vi "Finish.vi"   [LabVIEW 2013]
doc: "This VI is called just before exiting. It is expected to close I/O refnum, save collected data, etc."
uses:
  <vilib>/Rock Robotics/WPI/Joystick/WPI_JoystickGetSetRefNum.vi
types:
  T1 = typedef "WPI_MotorControlDeviceRef.ctl" = cluster{"DeviceStatus":errorcluster, "Type":enum16{"PWM", "CAN"}, "PWM":cluster{"Digital Module":T2, "PWM Channel":T3, "DeadBand":T4}, "CAN":cluster{"Device Number":u8, "Control Mode":T5, "Semaphore":T6, "Max Vout":dbl}, "Invert":bool, "TransformRef":T7, "InvTransformRef":T7}
  T2 = typedef "FPGA_TypedefDigitalModule.ctl" = enum16{"Digital Module 1", "Digital Module 2"}
  T3 = typedef "FPGA_DIOPWMChannel.ctl" = enum8{"PWM 1", "PWM 2", "PWM 3", "PWM 4", "PWM 5", "PWM 6", "PWM 7", "PWM 8", "PWM 9", "PWM 10", "Invalid"}
  T4 = typedef "WPI_PWMDeadband.ctl" = cluster{"Name":string, "maxPositivePwm":i32, "minPositivePwm":i32, "centerPwm":i32, "maxNegativePwm":i32, "minNegativePwm":i32, "angularRange":u16}
  T5 = typedef "WPI_CANJaguar_ControlMode.ctl" = enum8{"Percent VBus", "Current", "Speed", "Position", "Voltage"}
  T6 = typedef "Semaphore RefNum" = refnum<k1>
  T7 = typedef "WPI_PWMTransform_ConPane.ctl" = refnum<vi>
  T8 = typedef "WPI_SolenoidDevRef.ctl" = cluster{"DevStatus":errorcluster, "Solenoid Module":T9, "Forward Solenoid Channel":T10, "Reverse Solenoid Channel":T10}
  T9 = typedef "FPGA_TypedefSolenoidModule.ctl" = enum16{"Solenoid Module 1", "Solenoid Module 2"}
  T10 = typedef "WPI_SolenoidChannel.ctl" = enum8{"Solenoid 1", "Solenoid 2", "Solenoid 3", "Solenoid 4", "Solenoid 5", "Solenoid 6", "Solenoid 7", "Solenoid 8", "Invalid"}
  T11 = typedef "WPI_DigitalInputDevRef.ctl" = cluster{"DevStatus":errorcluster, "DIO Channel":T12, "Digital Module":T2}
  T12 = typedef "FPGA_DIOChannel.ctl" = enum8{"DIO 1", "DIO 2", "DIO 3", "DIO 4", "DIO 5", "DIO 6", "DIO 7", "DIO 8", "DIO 9", "DIO 10", "DIO 11", "DIO 12", "DIO 13", "DIO 14", "Invalid"}
  T13 = typedef "WPI_CameraDevRef.ctl" = cluster{"Camera Address":string, "CameraStatus":errorcluster, "Acquire Image Notifier":refnum<notifier>}
  T14 = typedef "WPI_JoystickDevRef.ctl" = cluster{"Device":T15}
  T15 = typedef "WPI_JoystickDeviceEnum.ctl" = enum16{"USB 1", "USB 2", "USB 3", "USB 4", "Kinect 1", "Kinect 2"}
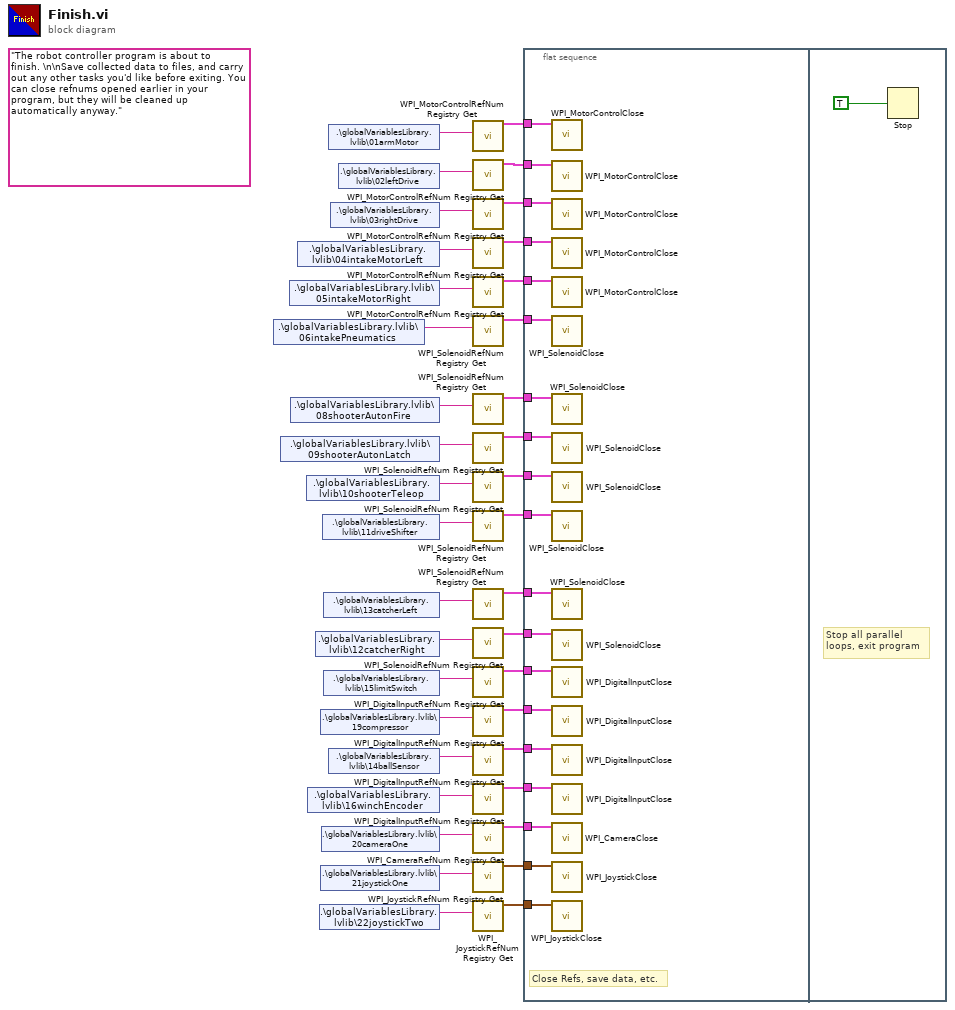
[diagram p0: block diagram]
diagram:
  (unwired) "The robot controller program is about to finish. \n\nSave collected data to files, and carry out any other tasks you'd like before exiting. You can close refnums opened earlier in your program, but they will be cleaned up automatically anyway."
  n1 = shared-variable ".\\globalVariablesLibrary.lvlib\\06intakePneumatics"() -> (w28:string)  [unwired: 1 in, 1 out]
  n2 = shared-variable ".\\globalVariablesLibrary.lvlib\\09shooterAutonLatch"() -> (w26:string)  [unwired: 1 in, 1 out]
  n3 = shared-variable ".\\globalVariablesLibrary.lvlib\\05intakeMotorRight"() -> (w34:string)  [unwired: 1 in, 1 out]
  n4 = shared-variable ".\\globalVariablesLibrary.lvlib\\08shooterAutonFire"() -> (w27:string)  [unwired: 1 in, 1 out]
  n5 = shared-variable ".\\globalVariablesLibrary.lvlib\\04intakeMotorLeft"() -> (w35:string)  [unwired: 1 in, 1 out]
  n6 = shared-variable ".\\globalVariablesLibrary.lvlib\\10shooterTeleop"() -> (w25:string)  [unwired: 1 in, 1 out]
  n7 = shared-variable ".\\globalVariablesLibrary.lvlib\\16winchEncoder"() -> (w11:string)  [unwired: 1 in, 1 out]
  n8 = shared-variable ".\\globalVariablesLibrary.lvlib\\12catcherRight"() -> (w22:string)  [unwired: 1 in, 1 out]
  n9 = shared-variable ".\\globalVariablesLibrary.lvlib\\22joystickTwo"() -> (w3:string)  [unwired: 1 in, 1 out]
  n10 = shared-variable ".\\globalVariablesLibrary.lvlib\\19compressor"() -> (w13:string)  [unwired: 1 in, 1 out]
  n11 = shared-variable ".\\globalVariablesLibrary.lvlib\\21joystickOne"() -> (w4:string)  [unwired: 1 in, 1 out]
  n12 = shared-variable ".\\globalVariablesLibrary.lvlib\\20cameraOne"() -> (w6:string)  [unwired: 1 in, 1 out]
  n13 = shared-variable ".\\globalVariablesLibrary.lvlib\\11driveShifter"() -> (w24:string)  [unwired: 1 in, 1 out]
  n14 = shared-variable ".\\globalVariablesLibrary.lvlib\\13catcherLeft"() -> (w23:string)  [unwired: 1 in, 1 out]
  n15 = shared-variable ".\\globalVariablesLibrary.lvlib\\15limitSwitch"() -> (w14:string)  [unwired: 1 in, 1 out]
  n16 = shared-variable ".\\globalVariablesLibrary.lvlib\\01armMotor"() -> (w38:string)  [unwired: 1 in, 1 out]
  n17 = shared-variable ".\\globalVariablesLibrary.lvlib\\14ballSensor"() -> (w12:string)  [unwired: 1 in, 1 out]
  n18 = shared-variable ".\\globalVariablesLibrary.lvlib\\03rightDrive"() -> (w36:string)  [unwired: 1 in, 1 out]
  n19 = shared-variable ".\\globalVariablesLibrary.lvlib\\02leftDrive"() -> (w37:string)  [unwired: 1 in, 1 out]
  n20 = call <vilib>:"WPI_MotorControlRefNum Registry Get.vi"("refnum name"=w38) -> ("MotorControlDevRef"=w33:T1)  [unwired: 9 in, 1 out]
  n21 = call <vilib>:"WPI_MotorControlRefNum Registry Get.vi"("refnum name"=w37) -> ("MotorControlDevRef"=w32:T1)  [unwired: 9 in, 1 out]
  n22 = call <vilib>:"WPI_MotorControlRefNum Registry Get.vi"("refnum name"=w36) -> ("MotorControlDevRef"=w31:T1)  [unwired: 9 in, 1 out]
  n23 = call <vilib>:"WPI_MotorControlRefNum Registry Get.vi"("refnum name"=w35) -> ("MotorControlDevRef"=w30:T1)  [unwired: 9 in, 1 out]
  n24 = call <vilib>:"WPI_MotorControlRefNum Registry Get.vi"("refnum name"=w34) -> ("MotorControlDevRef"=w29:T1)  [unwired: 9 in, 1 out]
  n25 = call <vilib>:"WPI_SolenoidRefNum Registry Get.vi"("refnum name"=w28) -> ("SolenoidDevRef"=w21:T8)  [unwired: 9 in, 1 out]
  n26 = call <vilib>:"WPI_SolenoidRefNum Registry Get.vi"("refnum name"=w27) -> ("SolenoidDevRef"=w20:T8)  [unwired: 9 in, 1 out]
  n27 = call <vilib>:"WPI_SolenoidRefNum Registry Get.vi"("refnum name"=w26) -> ("SolenoidDevRef"=w19:T8)  [unwired: 9 in, 1 out]
  n28 = call <vilib>:"WPI_SolenoidRefNum Registry Get.vi"("refnum name"=w25) -> ("SolenoidDevRef"=w18:T8)  [unwired: 9 in, 1 out]
  n29 = call <vilib>:"WPI_SolenoidRefNum Registry Get.vi"("refnum name"=w24) -> ("SolenoidDevRef"=w17:T8)  [unwired: 9 in, 1 out]
  n30 = call <vilib>:"WPI_SolenoidRefNum Registry Get.vi"("refnum name"=w23) -> ("SolenoidDevRef"=w16:T8)  [unwired: 9 in, 1 out]
  n31 = call <vilib>:"WPI_SolenoidRefNum Registry Get.vi"("refnum name"=w22) -> ("SolenoidDevRef"=w15:T8)  [unwired: 9 in, 1 out]
  n32 = call <vilib>:"WPI_DigitalInputRefNum Registry Get.vi"("refnum name"=w14) -> ("DigitalInputDevRef"=w10:T11)  [unwired: 9 in, 1 out]
  n33 = call <vilib>:"WPI_DigitalInputRefNum Registry Get.vi"("refnum name"=w13) -> ("DigitalInputDevRef"=w9:T11)  [unwired: 9 in, 1 out]
  n34 = call <vilib>:"WPI_DigitalInputRefNum Registry Get.vi"("refnum name"=w12) -> ("DigitalInputDevRef"=w8:T11)  [unwired: 9 in, 1 out]
  n35 = call <vilib>:"WPI_DigitalInputRefNum Registry Get.vi"("refnum name"=w11) -> ("DigitalInputDevRef"=w7:T11)  [unwired: 9 in, 1 out]
  n36 = call <vilib>:"WPI_CameraRefNum Registry Get.vi"("refnum name"=w6) -> ("CameraDevRef"=w5:T13)  [unwired: 9 in, 1 out]
  n37 = call <vilib>:"WPI_JoystickRefNum Registry Get.vi"("refnum name"=w4) -> ("JoystickDevRef"=w2:T14)  [unwired: 9 in, 1 out]
  n38 = call <vilib>:"WPI_JoystickRefNum Registry Get.vi"("refnum name"=w3) -> ("JoystickDevRef"=w1:T14)  [unwired: 9 in, 1 out]
  n39 = flat-sequence {
    tunnel: w33 -> [w57]
    tunnel: w32 -> [w56]
    tunnel: w31 -> [w55]
    tunnel: w30 -> [w54]
    tunnel: w29 -> [w53]
    tunnel: w21 -> [w52]
    tunnel: w20 -> [w51]
    tunnel: w19 -> [w50]
    tunnel: w18 -> [w49]
    tunnel: w17 -> [w48]
    tunnel: w16 -> [w47]
    tunnel: w15 -> [w46]
    tunnel: w10 -> [w45]
    tunnel: w9 -> [w44]
    tunnel: w8 -> [w43]
    tunnel: w7 -> [w42]
    tunnel: w5 -> [w41]
    tunnel: w2 -> [w40]
    tunnel: w1 -> [w39]
    frame #0 {
      # "Close Refs, save data, etc."
      n40 = call <vilib>:"WPI_MotorControlClose.vi"("MotorControlDevRef"=w57) -> ()  [unwired: 10 in, 1 out]
      n41 = call <vilib>:"WPI_MotorControlClose.vi"("MotorControlDevRef"=w56) -> ()  [unwired: 10 in, 1 out]
      n42 = call <vilib>:"WPI_MotorControlClose.vi"("MotorControlDevRef"=w55) -> ()  [unwired: 10 in, 1 out]
      n43 = call <vilib>:"WPI_MotorControlClose.vi"("MotorControlDevRef"=w54) -> ()  [unwired: 10 in, 1 out]
      n44 = call <vilib>:"WPI_MotorControlClose.vi"("MotorControlDevRef"=w53) -> ()  [unwired: 10 in, 1 out]
      n45 = call <vilib>:"WPI_SolenoidClose.vi"("SolenoidDevRef"=w52) -> ()  [unwired: 10 in, 1 out]
      n46 = call <vilib>:"WPI_SolenoidClose.vi"("SolenoidDevRef"=w51) -> ()  [unwired: 10 in, 1 out]
      n47 = call <vilib>:"WPI_SolenoidClose.vi"("SolenoidDevRef"=w50) -> ()  [unwired: 10 in, 1 out]
      n48 = call <vilib>:"WPI_SolenoidClose.vi"("SolenoidDevRef"=w49) -> ()  [unwired: 10 in, 1 out]
      n49 = call <vilib>:"WPI_SolenoidClose.vi"("SolenoidDevRef"=w48) -> ()  [unwired: 10 in, 1 out]
      n50 = call <vilib>:"WPI_SolenoidClose.vi"("SolenoidDevRef"=w47) -> ()  [unwired: 10 in, 1 out]
      n51 = call <vilib>:"WPI_SolenoidClose.vi"("SolenoidDevRef"=w46) -> ()  [unwired: 10 in, 1 out]
      n52 = call <vilib>:"WPI_DigitalInputClose.vi"("DigitalInputDevRef"=w45) -> ()  [unwired: 10 in, 1 out]
      n53 = call <vilib>:"WPI_DigitalInputClose.vi"("DigitalInputDevRef"=w44) -> ()  [unwired: 10 in, 1 out]
      n54 = call <vilib>:"WPI_DigitalInputClose.vi"("DigitalInputDevRef"=w43) -> ()  [unwired: 10 in, 1 out]
      n55 = call <vilib>:"WPI_DigitalInputClose.vi"("DigitalInputDevRef"=w42) -> ()  [unwired: 10 in, 1 out]
      n56 = call <vilib>:"WPI_CameraClose.vi"("CameraDevRef"=w41) -> ()  [unwired: 10 in, 1 out]
      n57 = call <vilib>:"WPI_JoystickClose.vi"("JoystickDevRef"=w40) -> ()  [unwired: 11 in]
      n58 = call <vilib>:"WPI_JoystickClose.vi"("JoystickDevRef"=w39) -> ()  [unwired: 11 in]
    }
    frame #1 {
      # "Stop all parallel\nloops, exit program"
      n59 = Stop(stop? (T)=TRUE ("Quit")) -> ()
    }
  }
